vi "Update.vi"(10 "Image":variant[][](array[variant]), 11 "Selection Views in":refnum<class "Graph with Section Views.lvclass">) -> (3 "Selection Views out":refnum<class "Graph with Section Views.lvclass">)   [LabVIEW 2023, in "Graph with Section Views.lvclass"]
uses:
  Graph with Section Views.lvclass
  Base Graph/Base Graph.lvclass/Base Graph.ctl
  Graph with Section Views.lvclass/Graph with Section Views.ctl
  Base Graph/Base Graph.lvclass
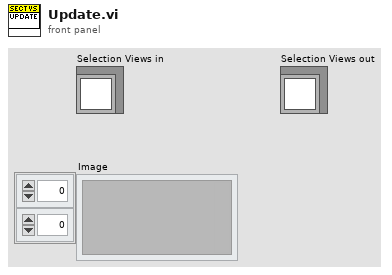
[diagram p1: front panel]
types:
  T1 = typedef "LVPointDoubleTypeDef.ctl" = cluster{"X":dbl, "Y":dbl}
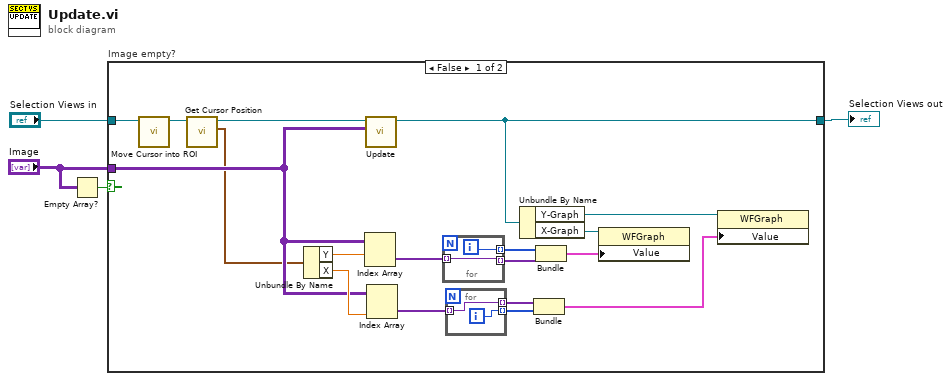
[diagram p0: block diagram]
diagram:
  n1 = Empty Array?(array="Image") -> (empty?=w2:bool)
  n2 = case "Image empty?" shown="False" w2 {
    tunnel: [w7 w27] -> w3
    tunnel: "Selection Views in" -> [w14 w27]
    tunnel: "Image" -> [w6 _]
    frame False {
      n3 = call "Move Cursor into ROI.vi"("Base Graph in"=w14) -> ("Base Graph out"=w9:refnum<class "Graph with Section Views.lvclass">)  [unwired: 10 in]
      n4 = call "Get Cursor Position.vi"("Base Graph in"=w9) -> ("Cursor Position"=w5:T1, "Base Graph out"=w8:refnum<class "Graph with Section Views.lvclass">)  [unwired: 9 in]
      n5 = Unbundle By Name(w5) -> ("Y"=w22:dbl, "X"=w21:dbl)
      n6 = Index Array(array=w6, index (row)=w22) -> (element=w11:variant[])  [unwired: 1 in]
      n7 = call-parent "Update.vi"("Image"=w6, "Base Graph in"=w8) -> ("Base Graph out"=w7:refnum<class "Graph with Section Views.lvclass">)  [unwired: 9 in]
      n8 = Index Array(array=w6, index (col)=w21) -> (element=w13:variant[])  [unwired: 1 in]
      n9 = for {
        tunnel: [w23] -> w15 mode=indexing
        tunnel: w11 -> [w24] mode=indexing
        tunnel: [w24] -> w10 mode=indexing
        i -> [w23]
      }
      n10 = for {
        tunnel: [w25] -> w20 mode=indexing
        tunnel: w13 -> [w26] mode=indexing
        tunnel: [w26] -> w12 mode=indexing
        i -> [w25]
      }
      n11 = Unbundle By Name(w7) -> ("Y-Graph"=w19:refnum<vi>, "X-Graph"=w18:refnum<vi>)
      n12 = Bundle(w12, w20) -> (w16:cluster{variant[], i32[]})  [unwired: 1 in]
      n13 = Bundle(w15, w10) -> (w17:cluster{i32[], variant[]})  [unwired: 1 in]
      n14 = property class="WFGraph"(reference=w18, "Value"=w17) -> ()  [unwired: 1 in, 2 out]
      n15 = property class="WFGraph"(reference=w19, "Value"=w16) -> ()  [unwired: 1 in, 2 out]
    }
    frame True {
    }
  }
  "Selection Views out" <- w3
